vi "Run.vi"(10 "API-Requests":T1, 11 "Actor in":refnum<class "Actor.lvclass">) -> (0 "error out":errorcluster, 3 "Actor out":refnum<class "Actor.lvclass">)   [LabVIEW 2018, in "Scripting.lvlib" / "Actor.lvlib" / "Actor.lvclass"]
uses:
  Actor.lvclass
  API-Requests.ctl
  Launch.ctl
  Stop.ctl
  Get State.ctl
  State.ctl
  Internal-Enqueuers.ctl
  Internal-Stop.ctl
  Internal-Error.ctl
  Interface.lvclass
types:
  T1 = typedef "Scripting.lvlib/Actor.lvlib/Actor.lvclass/API-Requests.ctl" = refnum<event-registration>
  T2 = typedef "Scripting.lvlib/Actor.lvlib/Actor.lvclass/Internal-Enqueuers.ctl" = cluster{"Stop":refnum<user-event>, "Error":refnum<user-event>}
  T3 = cluster{"API-Requests":T1, "Internal-Launch":refnum<event-registration>, "Internal-Stop":refnum<event-registration>, "Internal-Error":refnum<event-registration>}
  T4 = typedef "Scripting.lvlib/Actor.lvlib/Interface.lvclass/State.ctl" = cluster{"Current State":refnum<class "Actor.lvclass">}
  T5 = typedef "Scripting.lvlib/Actor.lvlib/Actor.lvclass/Internal-Stop.ctl" = cluster{"Type":enum16{"Normal", "Emergency"}}
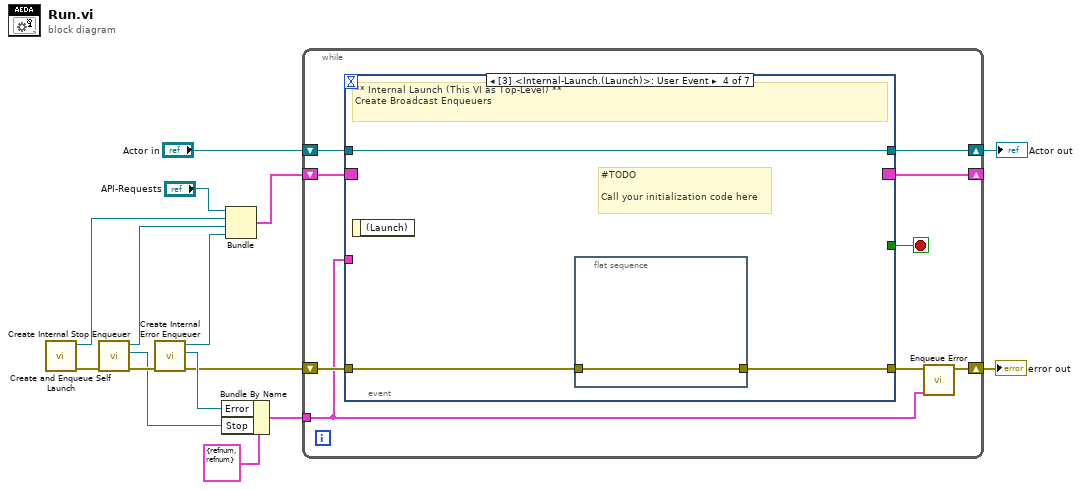
[diagram p0: block diagram]
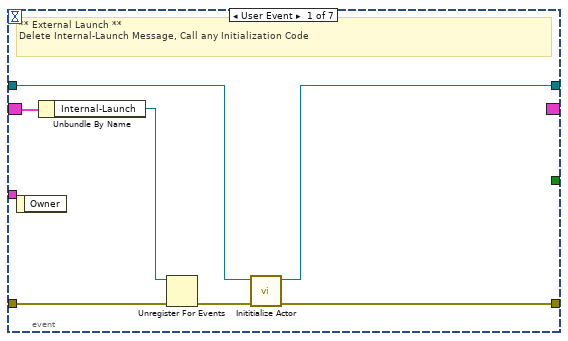
[diagram p2: hidden frame]
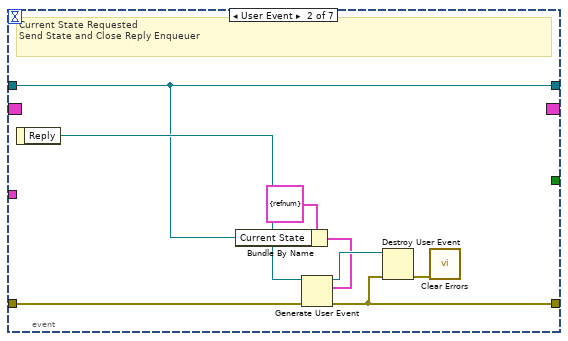
[diagram p3: hidden frame]
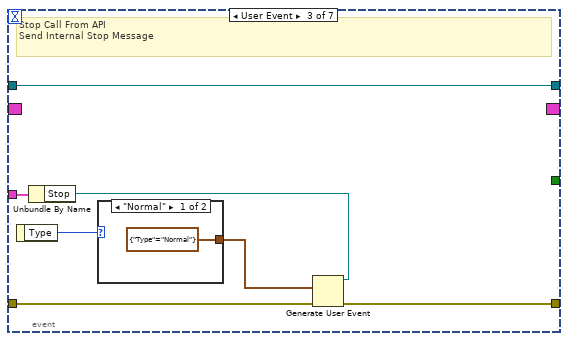
[diagram p4: hidden frame]
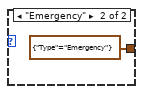
[diagram p5: hidden frame]
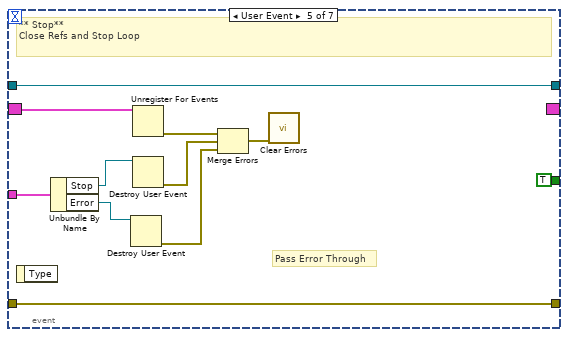
[diagram p6: hidden frame]
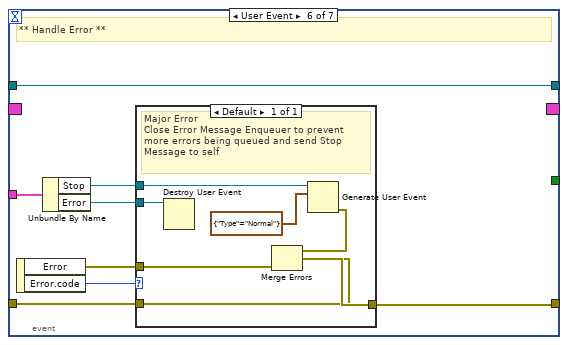
[diagram p7: hidden frame]
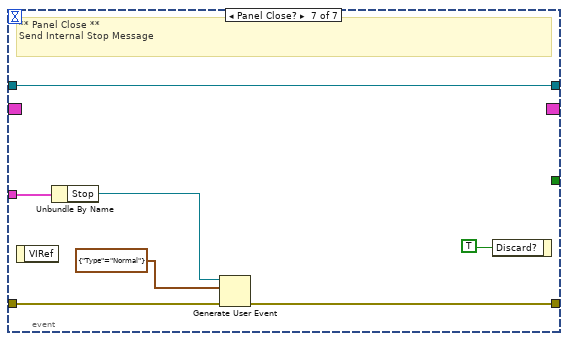
[diagram p8: hidden frame]
diagram:
  n1 = call "Create and Enqueue Self Launch.vi"() -> ("error out"=w12:errorcluster, "Internal-Launch"=w7:refnum<event-registration>)  [unwired: 10 in]
  n2 = call "Create Internal Stop Enqueuer.vi"("error in (no error)"=w12) -> ("error out"=w11:errorcluster, "Stop Enqueuer"=w9:refnum<user-event>, "Internal-Stop"=w6:refnum<event-registration>)  [unwired: 8 in]
  n3 = call "Create Internal Error Enqueuer.vi"("error in (no error)"=w11) -> ("error out"=w3:errorcluster, "Error Enqueuer"=w8:refnum<user-event>, "Internal-Error"=w5:refnum<event-registration>)  [unwired: 8 in]
  n4 = Bundle By Name(cluster=T2 {"Stop"=refnum, "Error"=refnum} ("States"), "Error"=w8, "Stop"=w9) -> (w2:T2)
  n5 = Bundle("API-Requests"="API-Requests", "Internal-Launch"=w7, "Internal-Stop"=w6, "Internal-Error"=w5) -> (w4:T3)  [unwired: 1 in]
  n6 = while {
    shift-right: [w22] -> w14
    shift-left: "Actor in" -> [w24]
    shift-right: [w19] -> w13
    shift-left: w3 -> [w23]
    shift-right: [w18] -> _
    shift-left: w4 -> [w17]
    tunnel: w2 -> [w16]
    stop <- w21 stop-if-true
    n7 = event shown="[3] <Internal-Launch.(Launch)>: User Event" {
      selector: w17 -> [w29 _ _ _ w59 _ _]
      dyn-events: [_ _ _ _ _ _ _] -> w18
      timeout: _ -> [_ _ _ _ _ _ _]
      tunnel: w24 -> [w27 w34 w46 w51 w63 w71 w85]
      tunnel: w23 -> [w30 w37 w45 w49 w62 w70 w83]
      tunnel: [w26 w34 w46 w51 w63 w71 w85] -> w22
      tunnel: [w25 w32 w44 w50 w62 w68 w82] -> w20
      tunnel: [_ _ _ _ TRUE _ _] -> w21
      tunnel: w16 -> [_ _ w42 _ w58 w65 w80]
      event User Event {
        # "** External Launch **\nDelete Internal-Launch Message, Call any Initialization Code"
        n8 = event-data() -> ()  [unwired: 1 in, 1 out]
        n9 = Unbundle By Name(w29) -> ("Internal-Launch"=w31:refnum<event-registration>)
        n10 = Unregister For Events(event registration refnum=w31, error in=w30) -> (error out=w28:errorcluster)
        n11 = call "Inititialize Actor.vi"("error in (no error)"=w28, "Actor in"=w27) -> ("error out"=w25:errorcluster, "Actor out"=w26:refnum<class "Actor.lvclass">)  [unwired: 8 in]
      }
      event User Event {
        # "Current State Requested\nSend State and Close Reply Enqueuer"
        n12 = event-data() -> ("Reply"=w39:refnum<user-event>)  [unwired: 1 in]
        n13 = Bundle By Name(cluster=T4 {"Current State"=refnum} ("event data"), "Current State"=w34) -> (w35:T4)
        n14 = Generate User Event(user event=w39, event data cluster=w35, error in=w37) -> (user event out=w36:refnum<user-event>, error out=w32:errorcluster)  [unwired: 1 in]
        n15 = Destroy User Event(user event=w36, error in=w32) -> (error out=w33:errorcluster)
        n16 = call <vilib>:"Clear Errors.vi"("error in (no error)"=w33) -> ()  [unwired: 5 in, 2 out]
      }
      event User Event {
        # "Stop Call From API\nSend Internal Stop Message"
        n17 = event-data() -> ("Type"=w43:enum16{"Normal", "Emergency"})  [unwired: 1 in]
        n18 = Unbundle By Name(w42) -> ("Stop"=w41:refnum<user-event>)
        n19 = case shown="\"Normal\"" w43 {
          tunnel: [T5 {"Type"=enum."Normal"} ("event data") T5 {"Type"=enum."Emergency"} ("event data")] -> w40
          frame "Normal" {
          }
          frame "Emergency" {
          }
        }
        n20 = Generate User Event(user event=w41, event data cluster=w40, error in=w45) -> (error out=w44:errorcluster)  [unwired: 1 in, 1 out]
      }
      event User Event {
        # "#TODO\n\nCall your initialization code here"
        # "** Internal Launch (This VI as Top-Level) **\nCreate Broadcast Enqueuers"
        n21 = event-data() -> ()  [unwired: 1 in, 1 out]
        n22 = flat-sequence {
          tunnel: w49 -> [w52]
          tunnel: [w52] -> w50
          frame #0 {
          }
        }
      }
      event User Event {
        # "Pass Error Through"
        # "** Stop**\nClose Refs and Stop Loop"
        n23 = event-data() -> ()  [unwired: 1 in, 1 out]
        n24 = Unbundle By Name(w58) -> ("Stop"=w56:refnum<user-event>, "Error"=w54:refnum<user-event>)
        n25 = Destroy User Event(user event=w54) -> (error out=w53:errorcluster)  [unwired: 1 in]
        n26 = Unregister For Events(event registration refnum=w59) -> (error out=w60:errorcluster)  [unwired: 1 in]
        n27 = Destroy User Event(user event=w56) -> (error out=w55:errorcluster)  [unwired: 1 in]
        n28 = Merge Errors(w60, w55, w53) -> (w57:errorcluster)
        n29 = call <vilib>:"Clear Errors.vi"("error in (no error)"=w57) -> ()  [unwired: 5 in, 2 out]
      }
      event User Event {
        # "** Handle Error **"
        n30 = event-data() -> ("Error"=w66:errorcluster, "Error.code"=w67:i32)  [unwired: 1 in]
        n31 = Unbundle By Name(w65) -> ("Stop"=w69:refnum<user-event>, "Error"=w64:refnum<user-event>)
        n32 = case shown="Default" w67 {
          tunnel: w70 -> [w75]
          tunnel: w69 -> [w73]
          tunnel: [w78] -> w68
          tunnel: w66 -> [w74]
          tunnel: w64 -> [w72]
          frame Default {
            # "Major Error\nClose Error Message Enqueuer to prevent more errors being queued and send Stop Message to self"
            n33 = Destroy User Event(user event=w72) -> ()  [unwired: 1 in, 1 out]
            n34 = Generate User Event(user event=w73, event data cluster=T5 {"Type"=enum."Normal"} ("event data")) -> (error out=w77:errorcluster)  [unwired: 2 in, 1 out]
            n35 = Merge Errors(w77, w75, w74) -> (w78:errorcluster)
          }
        }
      }
      event Panel Close? {
        # "** Panel Close **\nSend Internal Stop Message"
        n36 = event-data() -> ()  [unwired: 1 in, 1 out]
        n37 = Unbundle By Name(w80) -> ("Stop"=w79:refnum<user-event>)
        n38 = Generate User Event(user event=w79, event data cluster=T5 {"Type"=enum."Normal"} ("event data"), error in=w83) -> (error out=w82:errorcluster)  [unwired: 1 in, 1 out]
        n39 = event-data("Discard?"=TRUE) -> ()  [unwired: 1 in, 1 out]
      }
    }
    n40 = call "Enqueue Error.vi"("Error-Enqueuer in"=w16, "error in (no error)"=w20) -> ("error out"=w19:errorcluster)  [unwired: 8 in, 1 out]
  }
  "Actor out" <- w14
  "error out" <- w13
